vi "Write Controls to Config File.vi"(6 "Child?":bool, 7 "section":string, 8 "Error In":errorcluster, 9 "ParentName":string, 10 "Ctl Refnum":refnum<vi>, 11 "refnum":T1) -> (0 "Error Out":errorcluster, 3 "refnum out":T1)   [LabVIEW 2018]
uses:
  <vilib>/Utility/config.llb/Config Data RefNum.ctl
  Hardware Mfg/Thorlabs Translation Stages/Controls/Translation Stage Cluster.ctl
  Controls/Translation Stage Types.ctl
  <vilib>/Utility/config.llb/Write Key (String).vi
  <vilib>/Utility/config.llb/Write Key (U32).vi
  <vilib>/Utility/config.llb/Write Key (Boolean).vi
  <vilib>/Utility/config.llb/Write Key (Double).vi
  <vilib>/Utility/config.llb/NI_LVConfig.lvlib
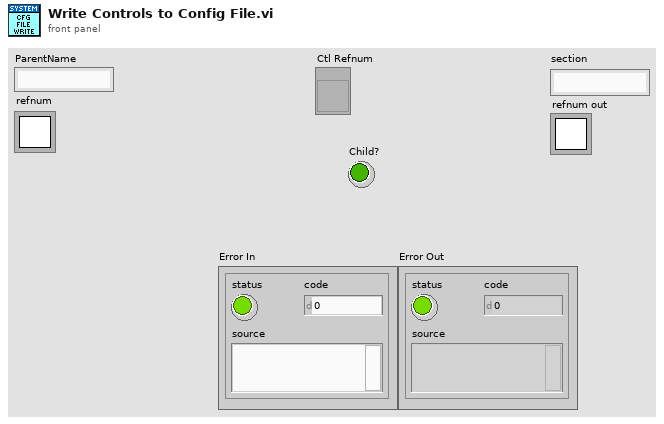
[diagram p1: front panel]
types:
  T1 = typedef "NI_LVConfig.lvlib/Config Data RefNum.ctl" = refnum<k1>
  T2 = typedef "Translation Stage Cluster.ctl" = cluster{"Position":dbl, "Is.Enabled?":bool, "Is.Connected?":bool, "Device SN":string, "AccelerationMaximum":dbl, "VelocityMaximum":dbl, "Acceleration":dbl, "Velocity":dbl, "waitTimeout (ms)":i32, "Model":T3, "Is.Homed?":bool, "MOVE":bool}
  T3 = typedef "Translation Stage Types.ctl" = enum16{"None", "Thorlabs LTS", "Thorlabs MLJ"}
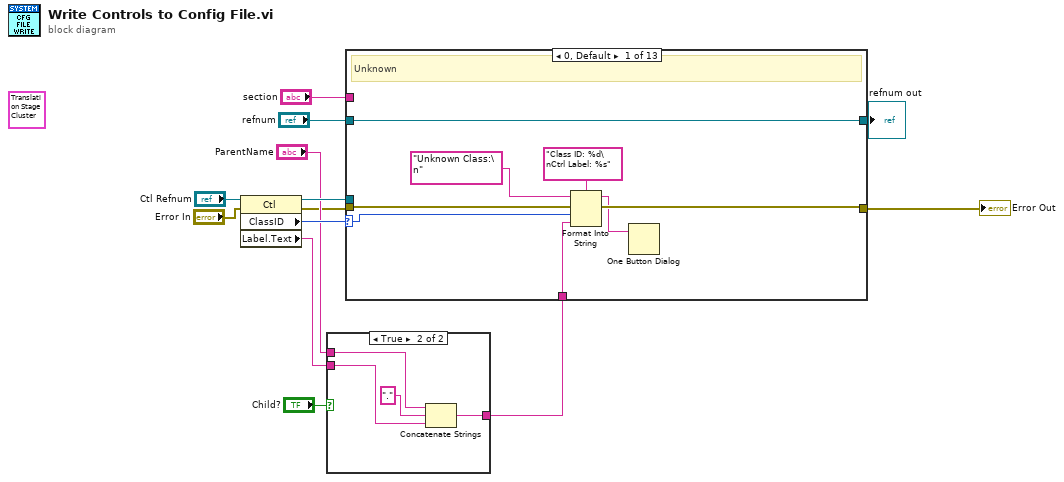
[diagram p0: block diagram]
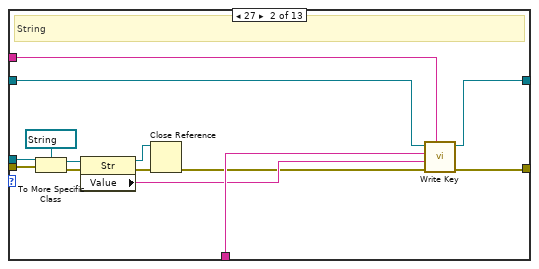
[diagram p3: hidden frame]
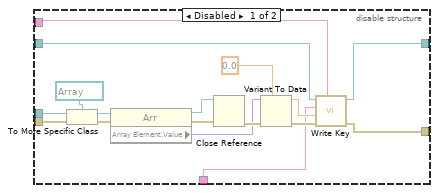
[diagram p5: hidden frame]
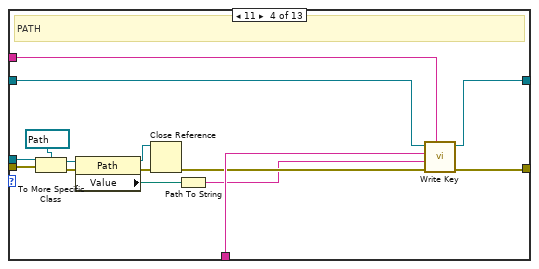
[diagram p6: hidden frame]
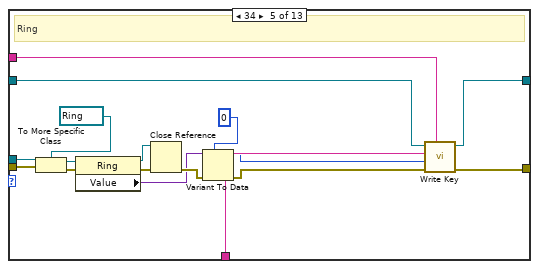
[diagram p7: hidden frame]
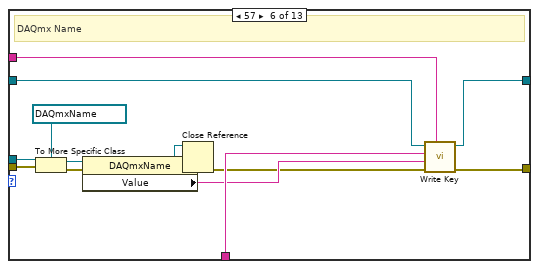
[diagram p8: hidden frame]
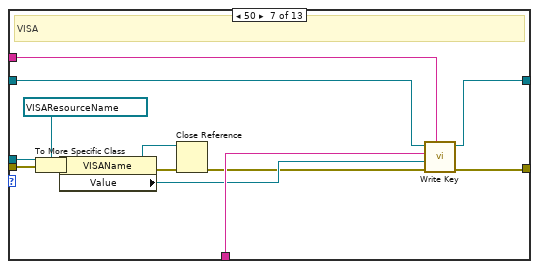
[diagram p9: hidden frame]
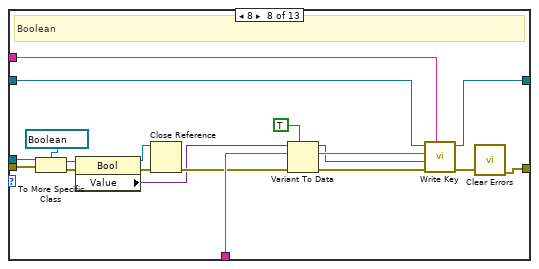
[diagram p10: hidden frame]
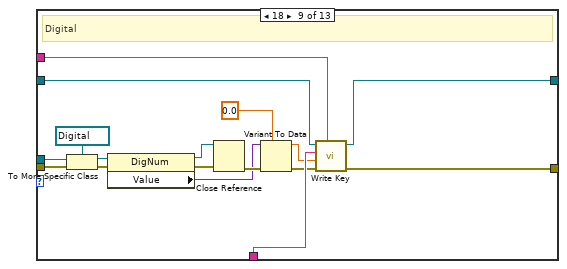
[diagram p11: hidden frame]
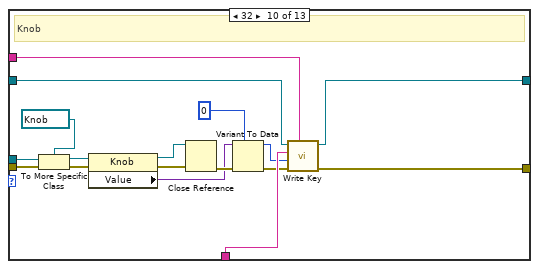
[diagram p12: hidden frame]
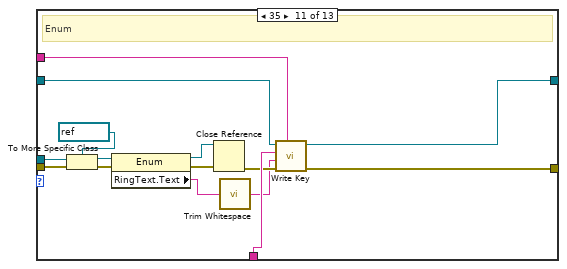
[diagram p13: hidden frame]
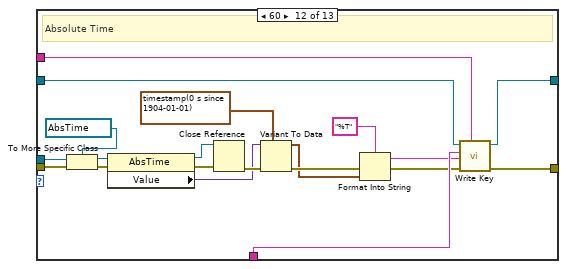
[diagram p14: hidden frame]
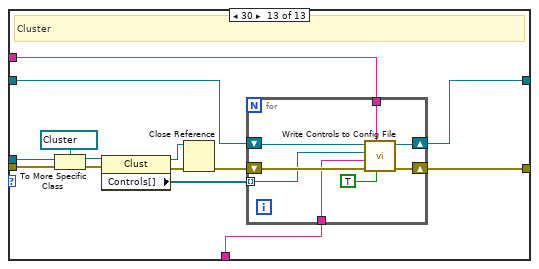
[diagram p15: hidden frame]
diagram:
  (unwired) T2 {"Position"=0.0, "Is.Enabled?"=FALSE, "Is.Connected?"=FALSE, "Device SN"="45876539", "AccelerationMaximum"=0.0, "VelocityMaximum"=0.0, "Acceleration"=0.0, "Velocity"=0.0, "waitTimeout (ms)"=0, "Model"=enum."None", "Is.Homed?"=FALSE, "MOVE"=FALSE} ("Control Param In")
  n1 = property class="Ctl"(reference="Ctl Refnum", error in="Error In") -> (reference out=w12:refnum<vi>, error out=w6:errorcluster, "ClassID"=w11:u32, "Label.Text"=w8:string)
  n2 = case shown="True" "Child?" {
    tunnel: "ParentName" -> [_ w18]
    tunnel: w8 -> [w14 w16]
    tunnel: [w14 w15] -> w3
    frame False {
    }
    frame True {
      n3 = Concatenate Strings(w18, ".", w16) -> (w15:string)
    }
  }
  n4 = case shown="0, Default" w11 {
    selector: w11 -> [w23 _ _ _ _ _ _ _ _ _ _ _ _]
    tunnel: w6 -> [w21 w39 w47 w80 w98 w112 w126 w143 w161 w178 w193 w213 w227]
    tunnel: w12 -> [_ w38 w46 w79 w97 w111 w125 w142 w160 w177 w192 w212 w225]
    tunnel: [w20 w37 w42 w78 w96 w110 w124 w127 w149 w167 w183 w202 w221] -> w1
    tunnel: "section" -> [_ w36 w45 w77 w95 w109 w123 w141 w152 w170 w186 w205 w218]
    tunnel: "refnum" -> [w26 w35 w44 w76 w94 w108 w122 w140 w151 w169 w185 w204 w220]
    tunnel: [w26 w34 w41 w75 w93 w107 w121 w139 w150 w168 w184 w203 w219] -> w2
    tunnel: w3 -> [w22 w32 w43 w73 w91 w105 w119 w137 w153 w171 w187 w206 w217]
    frame 0, Default {
      # "Unknown"
      n5 = Format Into String(format string="Class ID: %d\nCtrl Label: %s", initial string="Unknown Class:\n" ("string"), error in=w21, w23, w22) -> (resulting string=w19:string, error out=w20:errorcluster)
      n6 = One Button Dialog(message=w19) -> ()  [unwired: 1 in, 1 out]
    }
    frame 27 {
      # "String"
      n7 = To More Specific Class(target class=refnum<vi> refnum ("AccelerationMaximum 2"), reference=w38, error in=w39) -> (specific class reference=w30:refnum<vi>, error out=w33:errorcluster)
      n8 = property class="Str"(reference=w30, error in=w33) -> (reference out=w27:refnum<vi>, error out=w31:errorcluster, "Value"=w29:string)
      n9 = Close Reference(reference=w27, error in (no error)=w31) -> (error out=w28:errorcluster)
      n10 = call-poly <vilib>:"Write Key.vi"("section"=w36, "error in (no error)"=w28, "value"=w29, "key"=w32, "refnum"=w35) -> ("error out"=w37:errorcluster, "refnum out"=w34:T1)  [unwired: 4 in, 1 out]
    }
    frame 14 {
      n11 = disable-structure shown="Enabled" {
        disable-tunnel: w47 -> [w54 w66]
        disable-tunnel: w46 -> [w53 _]
        disable-tunnel: w45 -> [w52 _]
        disable-tunnel: w44 -> [w51 w65]
        disable-tunnel: w43 -> [w50 _]
        disable-tunnel: [w49 w66] -> w42
        disable-tunnel: [w48 w65] -> w41
        frame Disabled {
          n12 = To More Specific Class(target class=refnum<vi> refnum ("AccelerationMaximum 2"), reference=w53, error in=w54) -> (specific class reference=w62:refnum<vi>, error out=w63:errorcluster)
          n13 = property class="Arr"(reference=w62, error in=w63) -> (reference out=w60:refnum<vi>, error out=w61:errorcluster, "Array Element.Value"=w57:variant)
          n14 = Close Reference(reference=w60, error in (no error)=w61) -> (error out=w59:errorcluster)
          n15 = Variant To Data(error in=w59, type=0.0, Variant=w57) -> (data=w55:dbl, error out=w58:errorcluster)
          n16 = call-poly <vilib>:"Write Key.vi"("section"=w52, "error in (no error)"=w58, "value"=w55, "key"=w50, "refnum"=w51) -> ("error out"=w49:errorcluster, "refnum out"=w48:T1)  [unwired: 4 in, 1 out]
        }
        frame Enabled {
        }
      }
    }
    frame 11 {
      # "PATH"
      n17 = To More Specific Class(target class=refnum<vi> refnum ("AccelerationMaximum 2"), reference=w79, error in=w80) -> (specific class reference=w71:refnum<vi>, error out=w74:errorcluster)
      n18 = property class="Path"(reference=w71, error in=w74) -> (reference out=w68:refnum<vi>, error out=w72:errorcluster, "Value"=w70:path)
      n19 = Close Reference(reference=w68, error in (no error)=w72) -> (error out=w69:errorcluster)
      n20 = Path To String(path=w70) -> (string=w67:string)
      n21 = call-poly <vilib>:"Write Key.vi"("section"=w77, "error in (no error)"=w69, "value"=w67, "key"=w73, "refnum"=w76) -> ("error out"=w78:errorcluster, "refnum out"=w75:T1)  [unwired: 4 in, 1 out]
    }
    frame 34 {
      # "Ring"
      n22 = To More Specific Class(target class=refnum<vi> refnum ("Trigger Operation"), reference=w97, error in=w98) -> (specific class reference=w89:refnum<vi>, error out=w92:errorcluster)
      n23 = property class="Ring"(reference=w89, error in=w92) -> (reference out=w88:refnum<vi>, error out=w90:errorcluster, "Value"=w84:variant)
      n24 = Close Reference(reference=w88, error in (no error)=w90) -> (error out=w86:errorcluster)
      n25 = Variant To Data(error in=w86, type=u32 0, Variant=w84) -> (data=w82:u32, error out=w85:errorcluster)
      n26 = call-poly <vilib>:"Write Key.vi"("section"=w95, "error in (no error)"=w85, "value"=w82, "key"=w91, "refnum"=w94) -> ("error out"=w96:errorcluster, "refnum out"=w93:T1)  [unwired: 4 in, 1 out]
    }
    frame 57 {
      # "DAQmx Name"
      n27 = To More Specific Class(target class=refnum<vi> refnum ("Analog Out Channel"), reference=w111, error in=w112) -> (specific class reference=w103:refnum<vi>, error out=w106:errorcluster)
      n28 = property class="DAQmxName"(reference=w103, error in=w106) -> (reference out=w100:refnum<vi>, error out=w104:errorcluster, "Value"=w102:string)
      n29 = Close Reference(reference=w100, error in (no error)=w104) -> (error out=w101:errorcluster)
      n30 = call-poly <vilib>:"Write Key.vi"("section"=w109, "error in (no error)"=w101, "value"=w102, "key"=w105, "refnum"=w108) -> ("error out"=w110:errorcluster, "refnum out"=w107:T1)  [unwired: 4 in, 1 out]
    }
    frame 50 {
      # "VISA"
      n31 = To More Specific Class(target class=refnum<vi> refnum ("Controller VISA Ref"), reference=w125, error in=w126) -> (specific class reference=w117:refnum<vi>, error out=w120:errorcluster)
      n32 = property class="VISAName"(reference=w117, error in=w120) -> (reference out=w114:refnum<vi>, error out=w118:errorcluster, "Value"=w116:refnum<visa-resource-name>)
      n33 = Close Reference(reference=w114, error in (no error)=w118) -> (error out=w115:errorcluster)
      n34 = call-poly <vilib>:"Write Key.vi"("section"=w123, "error in (no error)"=w115, "value"=w116, "key"=w119, "refnum"=w122) -> ("error out"=w124:errorcluster, "refnum out"=w121:T1)  [unwired: 4 in, 1 out]
    }
    frame 8 {
      # "Boolean"
      n35 = To More Specific Class(target class=refnum<vi> refnum ("AccelerationMaximum 2"), reference=w142, error in=w143) -> (specific class reference=w135:refnum<vi>, error out=w138:errorcluster)
      n36 = property class="Bool"(reference=w135, error in=w138) -> (reference out=w133:refnum<vi>, error out=w136:errorcluster, "Value"=w131:variant)
      n37 = Close Reference(reference=w133, error in (no error)=w136) -> (error out=w134:errorcluster)
      n38 = Variant To Data(error in=w134, type=TRUE, Variant=w131) -> (data=w129:bool, error out=w132:errorcluster)
      n39 = call-poly <vilib>:"Write Key.vi"("section"=w141, "error in (no error)"=w132, "value"=w129, "key"=w137, "refnum"=w140) -> ("error out"=w128:errorcluster, "refnum out"=w139:T1)  [unwired: 4 in, 1 out]
      n40 = call <vilib>:"Clear Errors.vi"("error in (no error)"=w128) -> ("error out"=w127:errorcluster)  [unwired: 5 in, 1 out]
    }
    frame 18 {
      # "Digital"
      n41 = To More Specific Class(target class=refnum<vi> refnum ("AccelerationMaximum 2"), reference=w160, error in=w161) -> (specific class reference=w157:refnum<vi>, error out=w158:errorcluster)
      n42 = property class="DigNum"(reference=w157, error in=w158) -> (reference out=w155:refnum<vi>, error out=w156:errorcluster, "Value"=w147:variant)
      n43 = Close Reference(reference=w155, error in (no error)=w156) -> (error out=w154:errorcluster)
      n44 = Variant To Data(error in=w154, type=0.0, Variant=w147) -> (data=w145:dbl, error out=w148:errorcluster)
      n45 = call-poly <vilib>:"Write Key.vi"("section"=w152, "error in (no error)"=w148, "value"=w145, "key"=w153, "refnum"=w151) -> ("error out"=w149:errorcluster, "refnum out"=w150:T1)  [unwired: 4 in, 1 out]
    }
    frame 32 {
      # "Knob"
      n46 = To More Specific Class(target class=refnum<vi> refnum ("Zoom Factor"), reference=w177, error in=w178) -> (specific class reference=w175:refnum<vi>, error out=w176:errorcluster)
      n47 = property class="Knob"(reference=w175, error in=w176) -> (reference out=w173:refnum<vi>, error out=w174:errorcluster, "Value"=w165:variant)
      n48 = Close Reference(reference=w173, error in (no error)=w174) -> (error out=w172:errorcluster)
      n49 = Variant To Data(error in=w172, type=u32 0, Variant=w165) -> (data=w163:u32, error out=w166:errorcluster)
      n50 = call-poly <vilib>:"Write Key.vi"("section"=w170, "error in (no error)"=w166, "value"=w163, "key"=w171, "refnum"=w169) -> ("error out"=w167:errorcluster, "refnum out"=w168:T1)  [unwired: 4 in, 1 out]
    }
    frame 35 {
      # "Enum"
      n51 = To More Specific Class(target class=refnum<vi> refnum ("Enum"), reference=w192, error in=w193) -> (specific class reference=w190:refnum<vi>, error out=w191:errorcluster)
      n52 = property class="Enum"(reference=w190, error in=w191) -> (reference out=w188:refnum<vi>, error out=w189:errorcluster, "RingText.Text"=w180:string)
      n53 = Close Reference(reference=w188, error in (no error)=w189) -> (error out=w181:errorcluster)
      n54 = call <vilib>:"Trim Whitespace.vi"("string"=w180) -> ("trimmed string"=w179:string)  [unwired: 1 in]
      n55 = call-poly <vilib>:"Write Key.vi"("section"=w186, "error in (no error)"=w181, "value"=w179, "key"=w187, "refnum"=w185) -> ("error out"=w183:errorcluster, "refnum out"=w184:T1)  [unwired: 4 in, 1 out]
    }
    frame 60 {
      # "Absolute Time"
      n56 = To More Specific Class(target class=refnum<vi> refnum ("AccelerationMaximum 2"), reference=w212, error in=w213) -> (specific class reference=w210:refnum<vi>, error out=w211:errorcluster)
      n57 = property class="AbsTime"(reference=w210, error in=w211) -> (reference out=w208:refnum<vi>, error out=w209:errorcluster, "Value"=w200:variant)
      n58 = Close Reference(reference=w208, error in (no error)=w209) -> (error out=w207:errorcluster)
      n59 = Variant To Data(error in=w207, type=timestamp(0 s since 1904-01-01), Variant=w200) -> (data=w194:timestamp, error out=w201:errorcluster)
      n60 = Format Into String(format string="%T", error in=w201, w194) -> (resulting string=w198:string, error out=w199:errorcluster)  [unwired: 1 in]
      n61 = call-poly <vilib>:"Write Key.vi"("section"=w205, "error in (no error)"=w199, "value"=w198, "key"=w206, "refnum"=w204) -> ("error out"=w202:errorcluster, "refnum out"=w203:T1)  [unwired: 4 in, 1 out]
    }
    frame 30 {
      # "Cluster"
      n62 = To More Specific Class(target class=refnum<vi> refnum ("Cluster Ref In"), reference=w225, error in=w227) -> (specific class reference=w223:refnum<vi>, error out=w224:errorcluster)
      n63 = property class="Clust"(reference=w223, error in=w224) -> (reference out=w215:refnum<vi>, error out=w222:errorcluster, "Controls[]"=w214:refnum<vi>[])
      n64 = Close Reference(reference=w215, error in (no error)=w222) -> (error out=w216:errorcluster)
      n65 = for {
        tunnel: w218 -> [w231]
        tunnel: w217 -> [w230]
        shift-right: [w234] -> w221
        shift-left: w216 -> [w235]
        shift-right: [w232] -> w219
        shift-left: w220 -> [w233]
        tunnel: w214 -> [w228] mode=indexing
        n66 = call "Write Controls to Config File.vi"("Child?"=TRUE, "section"=w231, "Error In"=w235, "ParentName"=w230, "Ctl Refnum"=w228, "refnum"=w233) -> ("Error Out"=w234:errorcluster, "refnum out"=w232:T1)  [unwired: 4 in]
      }
    }
  }
  "Error Out" <- w1
  "refnum out" <- w2
